vi "Create Plugin Timing.vi"(8 "Async Tx":refnum<class "Transfer Group Timing.lvclass">[](array[class]), 9 "Async Rx":refnum<class "Transfer Group Timing.lvclass">[](array[class]), 10 "Inline Tx":refnum<class "Transfer Group Timing.lvclass">[](array[class]), 11 "Inline Rx":refnum<class "Transfer Group Timing.lvclass">[](array[class])) -> (3 "Plugin Timing Bundle":refnum<class "Plugin Timing.lvclass">)   [LabVIEW 2017, in "DSF Core.lvlib" / "Plugin Timing.lvclass"]
uses:
  Plugin Timing.lvclass
  Transfer Group Timing.lvclass
  Plugin Timing.lvclass/Plugin Timing.ctl
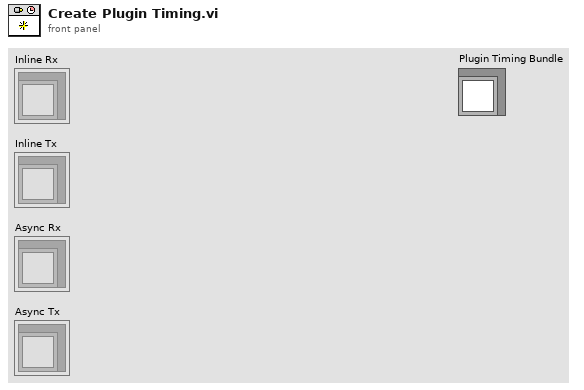
[diagram p1: front panel]
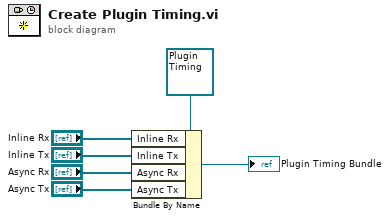
[diagram p0: block diagram]
diagram:
  n1 = Bundle By Name(cluster=refnum<class "Plugin Timing.lvclass"> refnum ("Plugin Timing in"), "Inline Rx"="Inline Rx", "Inline Tx"="Inline Tx", "Async Rx"="Async Rx", "Async Tx"="Async Tx") -> (→"Plugin Timing Bundle":refnum<class "Plugin Timing.lvclass">)
